vi "Add Step.vi"(7 "reset load":bool, 8 "input valid":bool, 10 "Data":T1, 11 "SegmentSequencer in":refnum<class "SegmentSequencer.lvclass">) -> (3 "SegmentSequencer out":refnum<class "SegmentSequencer.lvclass">)   [LabVIEW 2019, in "TX burst sequencer.lvlib" / "SegmentSequencer.lvclass"]
uses:
  SegmentSequencer.lvclass
  SegmentSequencer.lvclass/SegmentSequencer.ctl
  <vilib>/rvi/DataTransferAndStorage/Container/Common/niFpgaContainerExecOnDevCompGetState.vi
  <vilib>/rvi/Emulation/niFpgaEmulationIsFPGAContextNoSignature.vi
  <vilib>/rvi/DataTransferAndStorage/Container/Common/niFpgaContainerGetUniqueNameForEmu.vi
  <vilib>/rvi/Memory/Memory_Emulation/niFpgaMemoryEmulationCacheClearOnFirstRun.vi
  <vilib>/rvi/Memory/Memory_Emulation/nirvimemoryEmulationManagerCache_MakeExclusive.vi
  <vilib>/rvi/Memory/Memory_Emulation/niFpgaMemoryEmulationValidateCache.vi
  <vilib>/rvi/Memory/Memory_Emulation/nirvimemoryEmulationManagerCache_InsertValue.vi
  <vilib>/Utility/error.llb/Clear Errors.vi
  <vilib>/rvi/Memory/Memory_Emulation/nirvimemoryEmulationManagerCache_ReleaseExclusive.vi
  <vilib>/rvi/Memory/Memory_Emulation/nirvimemoryEmulationManagerCache_GetValue.vi
  <vilib>/rvi/Memory/Memory_Emulation/nirvimemoryEmulationManagerCache_SetValue.vi
  <vilib>/rvi/Emulation/niFpgaProcessEmulError.vi
  <vilib>/rvi/Emulation/niFpgaSctlEmulationGetInTimedLoop.vi
  <vilib>/rvi/errors/nirviReportUnexpectedCaseInternalError (U32).vi
  <vilib>/rvi/Emulation/niFpgaSctlEmulationResourceMgr.vi
  <vilib>/rvi/DataTransferAndStorage/Container/XNode/niFpgaContainer.xnode
  <vilib>/rvi/DataTransferAndStorage/Register/Emulation/niFpgaRegisterEmulationRefIn.vi
  <vilib>/rvi/Memory/Memory_Emulation/niFpgaMemoryEmulationRefIn.vi
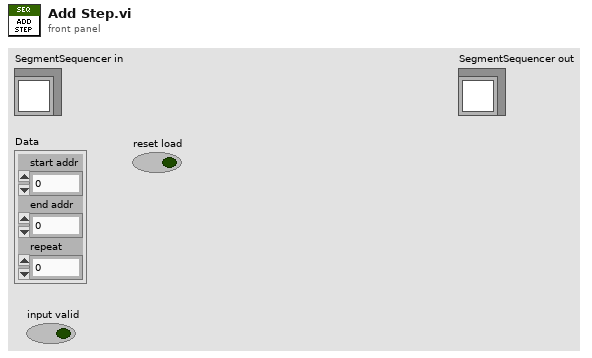
[diagram p1: front panel]
types:
  T1 = cluster{"start addr":u32, "end addr":u32, "repeat":u64}
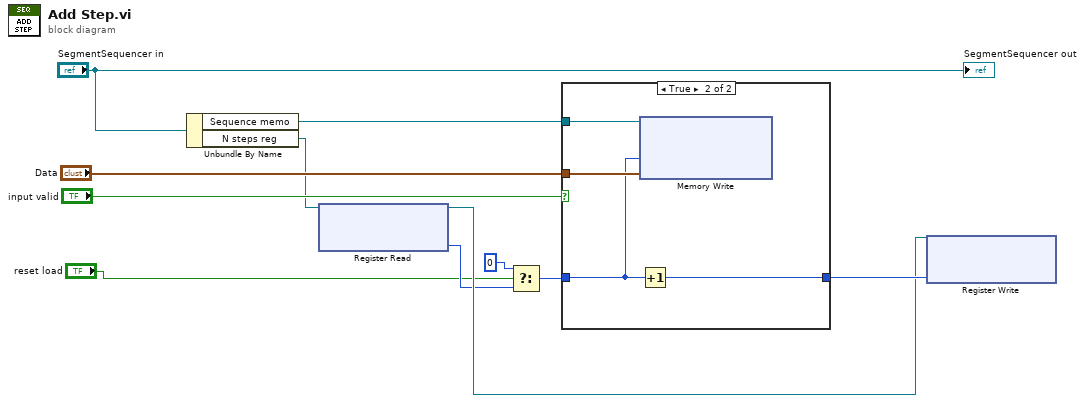
[diagram p0: block diagram]
diagram:
  n1 = Unbundle By Name("SegmentSequencer in") -> ("Sequence memo"=w7:refnum<k21>, "N steps reg"=w6:refnum<k21>)
  n2 = xnode ("Register Read")("Register In"=w6) -> ("Data"=w4:u32, "Register Out"=w5:refnum<k21>)
  n3 = Select(t=u32 0, s="reset load", f=w4) -> (s? t:f=w1:u32)
  n4 = case shown="True" "input valid" {
    tunnel: "Data" -> [_ w16]
    tunnel: [w12 w15] -> w8
    tunnel: w7 -> [_ w14]
    tunnel: w1 -> [w12 w13]
    frame False {
    }
    frame True {
      n5 = xnode ("Memory Write")("Address"=w13, "Data"=w16, "Memory In"=w14) -> ()  [unwired: 1 out]
      n6 = Increment(x=w13) -> (x+1=w15:u32)
    }
  }
  n7 = xnode ("Register Write")("Data"=w8, "Register In"=w5) -> ()  [unwired: 1 out]
  "SegmentSequencer out" <- "SegmentSequencer in"
